vi "SelectClosestPoint.vi"(1 "Mouse Position":cluster{"X":i32, "Y":i32}, 2 "Points":cluster{"Edge Info":T1, "Boolean":bool}[](array[cluster]) {"Edge Info"."Distance (Real-World)" format="%.2f"; "Edge Info"."Location (Real-World)"."Y" format="%.2g"; "Edge Info"."Location (Real-World)"."X" format="%.2f"; "Edge Info"."Noise" format="%.2f"; "Edge Info"."Location (Pixel)"."Y" format="%.2g"; "Edge Info"."Location (Pixel)"."X" format="%.2f"; "Edge Info"."Strength" format="%.2f"; "Edge Info"."Distance (Pixel)" format="%.2f"}) -> (0 "Point index":i32)   [LabVIEW 2014]
uses:
  <vilib>/vision/NI_Vision_Development_Module.lvlib
  <vilib>/vision/Measure.llb/Edge New.ctl
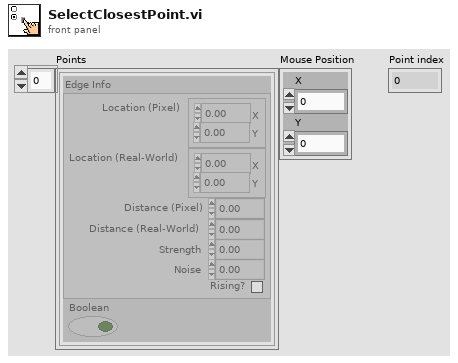
[diagram p1: front panel]
types:
  T1 = typedef "Edge New.ctl" = cluster{"Location (Pixel)":cluster{"X":sgl, "Y":sgl}, "Location (Real-World)":cluster{"X":sgl, "Y":sgl}, "Distance (Pixel)":dbl, "Distance (Real-World)":dbl, "Strength":dbl, "Noise":dbl, "Rising?":bool}
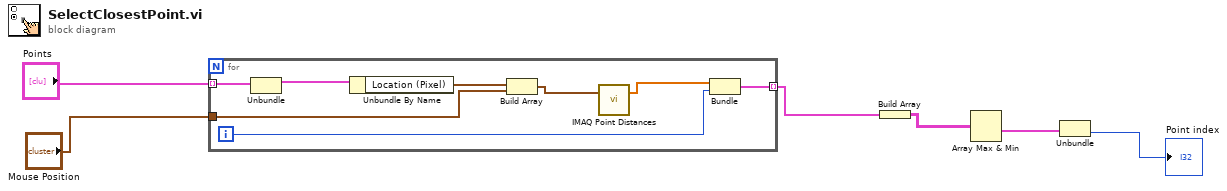
[diagram p0: block diagram]
diagram:
  n1 = for {
    tunnel: "Points" -> [w14] mode=indexing
    tunnel: "Mouse Position" -> [w12]
    tunnel: [w9] -> w1 mode=indexing
    i -> [w7]
    n2 = Unbundle(w14) -> ("Edge Info"=w13:T1)  [unwired: 1 out]
    n3 = Unbundle By Name(w13) -> ("Location (Pixel)"=w11:cluster{"X":sgl, "Y":sgl})
    n4 = Build Array(w11, w12) -> (w10:cluster{"X":sgl, "Y":sgl}[])
    n5 = call "IMAQ Point Distances"("Points"=w10) -> ("Distances"=w8:sgl[])  [unwired: 4 in, 1 out]
    n6 = Bundle("Distances"=w8, w7) -> (w9:cluster{"Distances":sgl[], i32})  [unwired: 1 in]
  }
  n7 = Build Array(w1) -> (w2:cluster{"Distances":sgl[], i32}[][])
  n8 = Array Max & Min(array=w2) -> (min value=w6:cluster{"Distances":sgl[], i32})  [unwired: 3 out]
  n9 = Unbundle(w6) -> (→"Point index":i32)  [unwired: 1 out]
